vi "parse.series_id.from_comic.vi"(11 "comic":T1) -> (1 "series.name":string, 3 "series_id":string)   [LabVIEW 2024]
uses:
  TypeDefs/comic--cluster.ctl
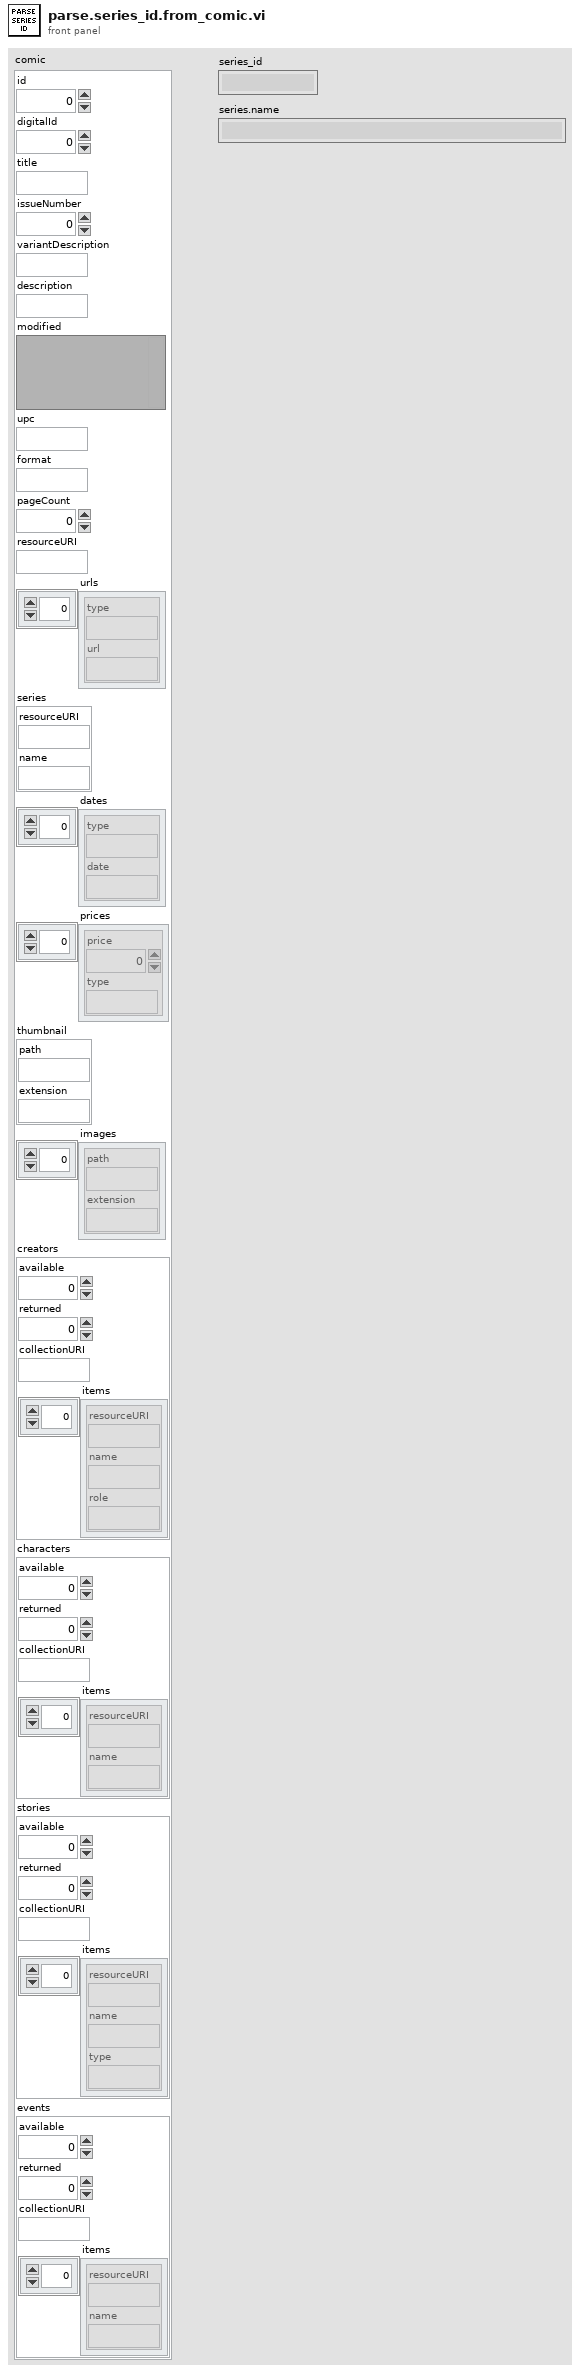
[diagram p1: front panel]
types:
  T1 = typedef "comic--cluster.ctl" = cluster{"id":i32, "digitalId":i32, "title":string, "issueNumber":i32, "variantDescription":string, "description":string, "modified":variant, "upc":string, "format":string, "pageCount":i32, "resourceURI":string, "urls":cluster{"type":string, "url":string}[], "series":cluster{"resourceURI":string, "name":string}, "dates":cluster{"type":string, "date":string}[], "prices":cluster{"price":dbl, "type":string}[], "thumbnail":cluster{"path":string, "extension":string}, "images":cluster{"path":string, "extension":string}[], "creators":cluster{"available":i32, "returned":i32, "collectionURI":string, "items":cluster{"resourceURI":string, "name":string, "role":string}[]}, "characters":cluster{"available":i32, "returned":i32, "collectionURI":string, "items":cluster{"resourceURI":string, "name":string}[]}, "stories":cluster{"available":i32, "returned":i32, "collectionURI":string, "items":cluster{"resourceURI":string, "name":string, "type":string}[]}, "events":cluster{"available":i32, "returned":i32, "collectionURI":string, "items":cluster{"resourceURI":string, "name":string}[]}}
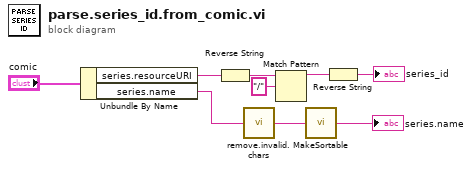
[diagram p0: block diagram]
diagram:
  n1 = Unbundle By Name("comic") -> ("series.resourceURI"=w8:string, "series.name"=w3:string)
  n2 = Reverse String(1:w8) -> (0:w7:string)
  n3 = call "remove.invalid.chars.vi"("string in"=w3) -> ("string out"=w2:string)
  n4 = Match Pattern(string=w7, regular expression="/") -> (before substring=w5:string)  [unwired: 1 in, 3 out]
  n5 = call "MakeSortable.vi"("string in"=w2) -> ("string out"=→"series.name":string)
  n6 = Reverse String(1:w5) -> (0:→"series_id":string)
